vi "Get LowLimit.vi"(8 "error in":errorcluster, 11 "Object Type in":refnum<class "Object Type Base.lvclass">) -> (0 "error out":errorcluster, 1 "Set?":bool, 2 "LowLimit":string, 3 "Object Type out":refnum<class "Object Type Base.lvclass">)   [LabVIEW 2024, in "Electronic Datasheet.lvlib" / "Object Type Base.lvclass"]
uses:
  Object Type Base.lvclass
  Object Type Base.lvclass/Object Type Base.ctl
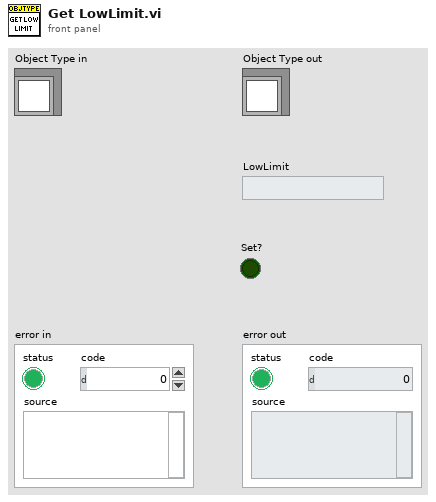
[diagram p1: front panel]
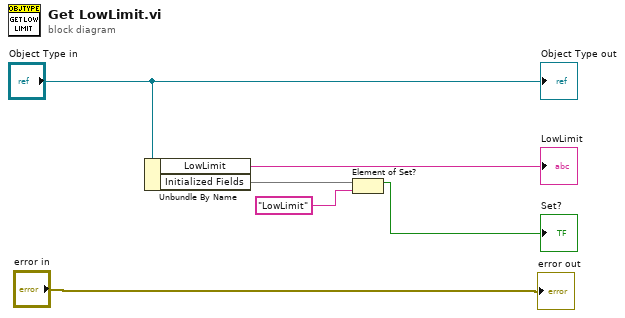
[diagram p0: block diagram]
diagram:
  n1 = Unbundle By Name("Object Type in") -> ("LowLimit"=→"LowLimit":string, "Initialized Fields"=w4:set{string})
  n2 = Element of Set?(10:"LowLimit" ("element"), 11:w4) -> (3:→"Set?":bool)
  "Object Type out" <- "Object Type in"
  "error out" <- "error in"
